vi "ErrorHandler.vi"(8 "error in (no error)":errorcluster, 11 "queue out":refnum<queue>) -> (0 "error out":errorcluster)   [LabVIEW 2019, in "Prueba08.lvclass"]
uses:
  Prueba08.lvclass
  MessageP08.ctl
  Controles/EstadosP08.ctl
  <vilib>/ErrorRing/Error Ring.xnode
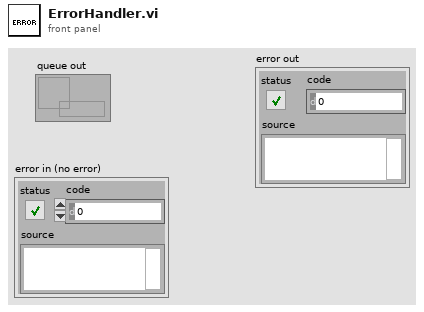
[diagram p1: front panel]
types:
  T1 = typedef "Prueba08.lvclass/EstadosP08.ctl" = enum16{"Error", "DetieneInstrumentos", "InicializarInstrumentos", "inicio", "configuraTabla", "FrecAmp1", "FrecAmp2", "nivelMaxRef", "iniciarGEN", "iniciarGEN_burst", "detenerGEN", "llenaTablaTemporal", "guardaVref", "monitoreo", "ingresaMediciones", "guardaMediciones", "cumplimiento", "listo_evaluar", "evaluar", "LeerArchivoConfiguracion", "final", "salir"}
  T2 = typedef "Prueba08.lvclass/MessageP08.ctl" = cluster{"Estados":T1, "Data":variant}
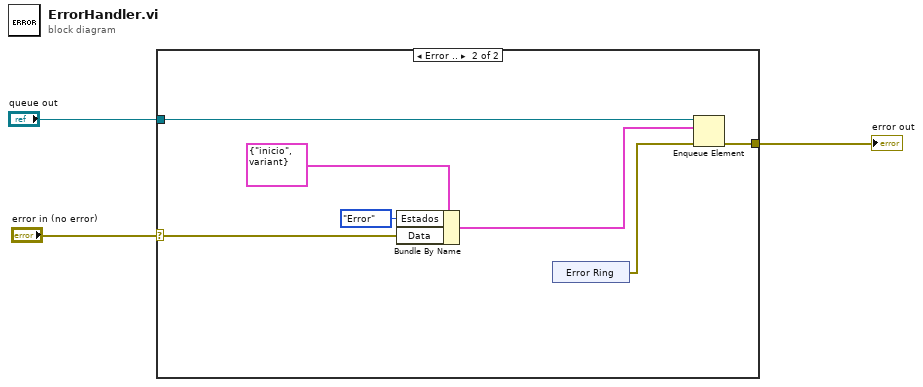
[diagram p0: block diagram]
diagram:
  n1 = case shown="Error .." "error in (no error)" {
    selector: "error in (no error)" -> [w4 w9]
    tunnel: "queue out" -> [_ w10]
    tunnel: [w4 w11] -> w2
    frame No Error {
    }
    frame Error {
      n2 = Bundle By Name(cluster=T2 {"Estados"=enum."inicio", "Data"=variant} ("MessageP08"), "Estados"=EstadosP08."Error", "Data"=w9) -> (w8:T2)
      n3 = xnode "Error Ring"() -> ("error out"=w7:errorcluster)
      n4 = Enqueue Element(queue=w10, element=w8, error in (no error)=w7) -> (error out=w11:errorcluster)  [unwired: 1 in, 2 out]
    }
  }
  "error out" <- w2
